vi "Move the pointer 2014.vi"(2 "error in (no error)":errorcluster, 3 "Servo Angles":cluster{"Angle X":dbl, "Angle Y":dbl}, 4 "Device In":i32) -> (0 "error out":errorcluster, 1 "Device Out":i32)   [LabVIEW 2014]
doc: "This vi will move the servos to the angles passed in radians to position the pointer."
panel:
  out "Y servo":dbl
  out "X servo":dbl
  out "Y degrees":dbl
  out "X degrees":dbl
  in  "Y zero":dbl=120.0
  in  "Y Gain":dbl=1.0
  in  "X zero":dbl=120.0
  in  "X Gain":dbl=1.0
  in  "Y Offset":dbl
  in  "X Offset":dbl
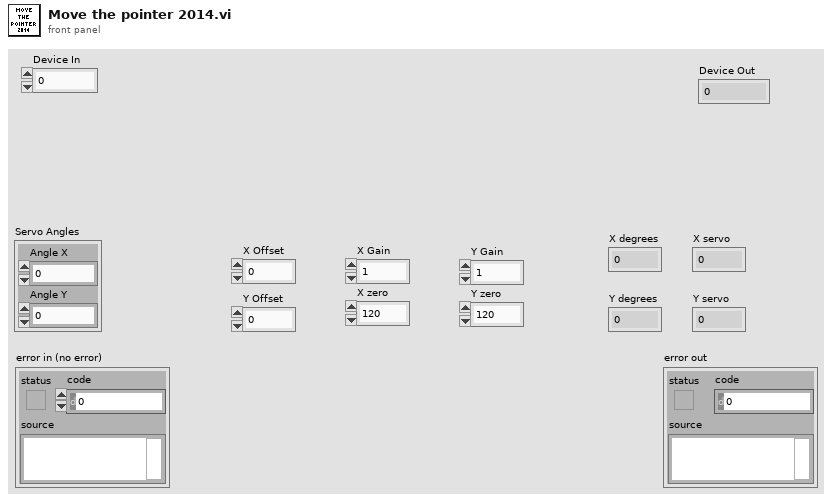
[diagram p1: front panel]
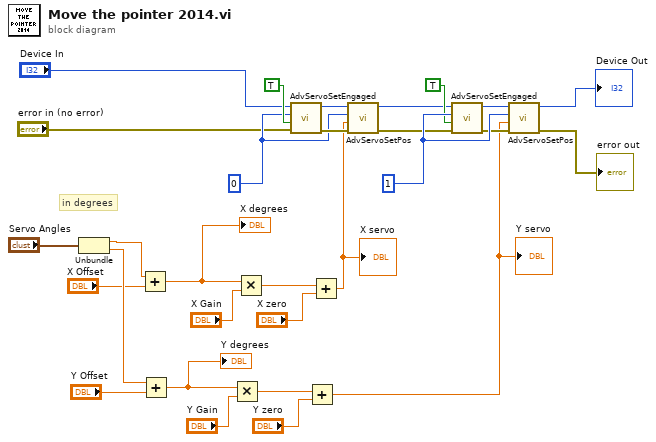
[diagram p0: block diagram]
diagram:
  w15 = 1
  w16 = 0
  # "in degrees"
  n1 = Unbundle("Servo Angles") -> ("Angle X"=w28:dbl, "Angle Y"=w27:dbl)
  n2 = Add(x=w28, y="X Offset") -> (x+y=w2:dbl)
  "X degrees" <- w2
  n3 = Add(x=w27, y="Y Offset") -> (x+y=w1:dbl)
  "Y degrees" <- w1
  n4 = Multiply(x=w1, y="Y Gain") -> (x*y=w21:dbl)
  n5 = Multiply(x=w2, y="X Gain") -> (x*y=w24:dbl)
  n6 = call "AdvServoSetEngaged.vi"("error in (no error)"="error in (no error)", "SetEngaged"=TRUE, "index"=w16, "Device In"="Device In") -> ("error out"=w17:errorcluster, "Device Out"=w18:i32)  [unwired: 5 in]
  n7 = Add(x=w21, y="Y zero") -> (x+y=w4:dbl)
  "Y servo" <- w4
  n8 = Add(x=w24, y="X zero") -> (x+y=w5:dbl)
  "X servo" <- w5
  n9 = call "AdvServoSetPos.vi"("error in (no error)"=w17, "pos_in"=w5, "index"=w16, "Device In"=w18) -> ("error out"=w10:errorcluster, "Device Out"=w11:i32)  [unwired: 5 in]
  n10 = call "AdvServoSetEngaged.vi"("error in (no error)"=w10, "SetEngaged"=TRUE, "index"=w15, "Device In"=w11) -> ("error out"=w14:errorcluster, "Device Out"=w13:i32)  [unwired: 5 in]
  n11 = call "AdvServoSetPos.vi"("error in (no error)"=w14, "pos_in"=w4, "index"=w15, "Device In"=w13) -> ("error out"=→"error out":errorcluster, "Device Out"=→"Device Out":i32)  [unwired: 5 in]
